vi "Lab 3 - Monty Hall - Copy (2).vi"() -> ()   [LabVIEW 2025]
panel:
  in  "Door 3":bool
  in  "Door 2":bool
  in  "Door 1":bool
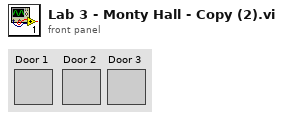
[diagram p1: front panel]
types:
  T1 = enum16{"Left Button", "Center Button", "Right Button", "Window Close"}
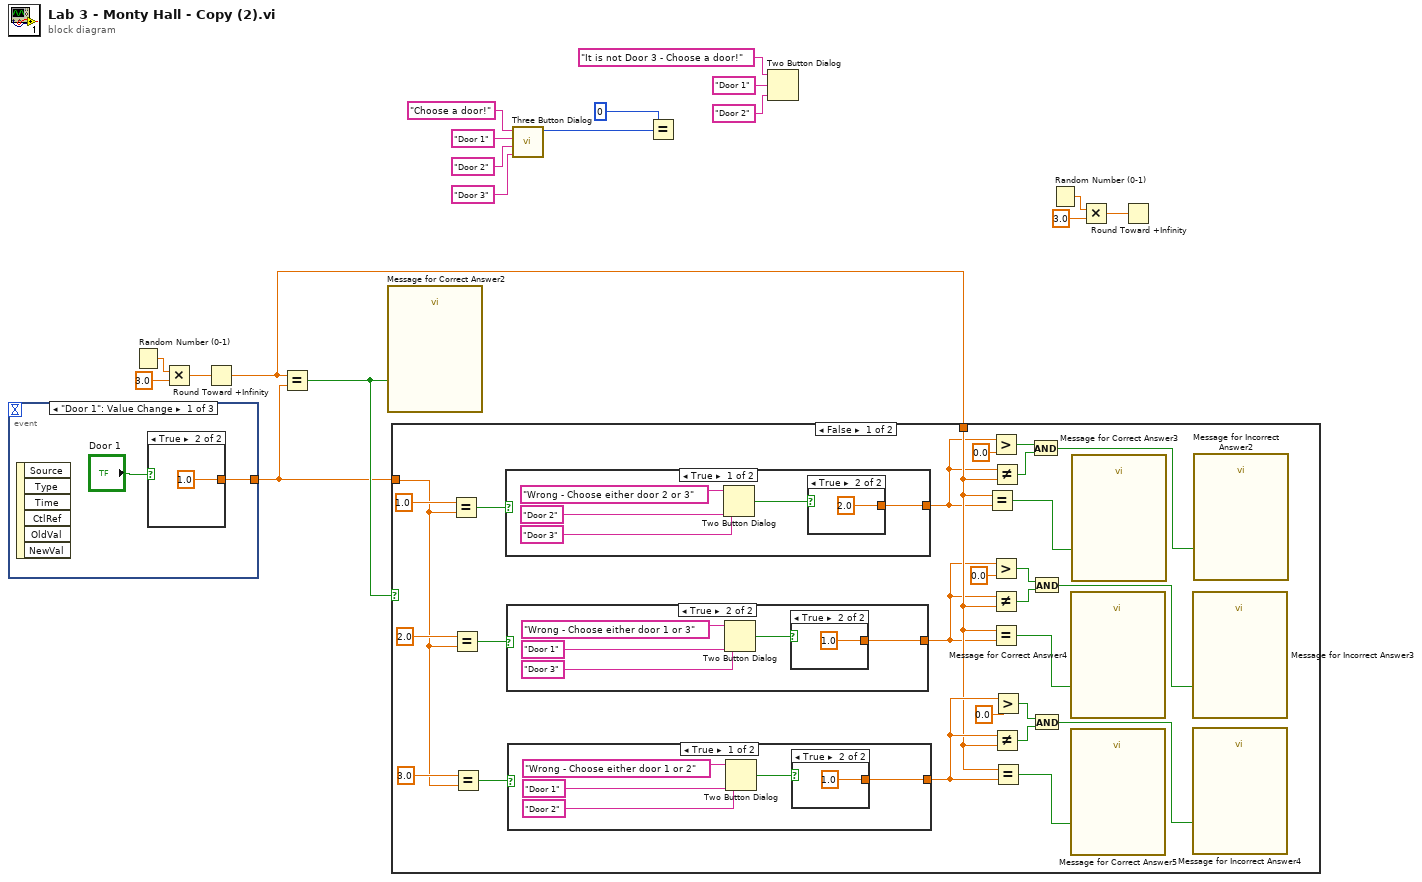
[diagram p0: block diagram]
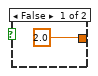
[diagram p2: hidden frame]
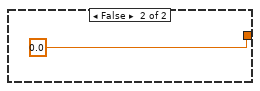
[diagram p3: hidden frame]
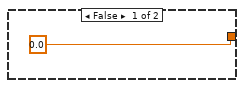
[diagram p4: hidden frame]
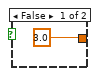
[diagram p5: hidden frame]
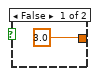
[diagram p6: hidden frame]
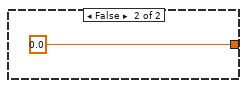
[diagram p7: hidden frame]
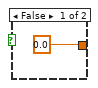
[diagram p9: hidden frame]
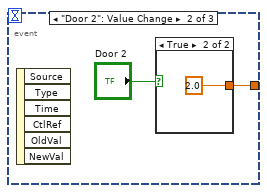
[diagram p10: hidden frame]
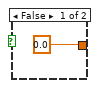
[diagram p11: hidden frame]
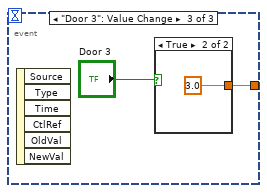
[diagram p12: hidden frame]
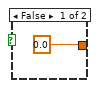
[diagram p13: hidden frame]
diagram:
  n1 = event shown="[0] \"Door 1\": Value Change" {
    selector: _ -> [_ _ _]
    dyn-events: _ -> [_ _ _]
    timeout: _ -> [_ _ _]
    tunnel: [w19 w23 w27] -> w15
    event "Door 1": Value Change {
      n2 = event-data() -> ()  [unwired: 1 in, 6 out]
      n3 = case shown="True" "Door 1" {
        tunnel: [0.0 1.0] -> w19
        frame False {
        }
        frame True {
        }
      }
    }
    event "Door 2": Value Change {
      n4 = event-data() -> ()  [unwired: 1 in, 6 out]
      n5 = case shown="True" "Door 2" {
        tunnel: [0.0 2.0] -> w23
        frame False {
        }
        frame True {
        }
      }
    }
    event "Door 3": Value Change {
      n6 = event-data() -> ()  [unwired: 1 in, 6 out]
      n7 = case shown="True" "Door 3" {
        tunnel: [0.0 3.0] -> w27
        frame False {
        }
        frame True {
        }
      }
    }
  }
  n8 = Random Number (0-1)() -> (number: 0 to 1=w17:dbl)
  n9 = Multiply(x=w17, y=3.0) -> (x*y=w14:dbl)
  n10 = Round Toward +Infinity(x=w14) -> (ceil(x): smallest int >= x=w13:dbl)
  n11 = Equal?(x=w13, y=w15) -> (x = y?=w16:bool)
  n12 = call "Message for Correct Answer2"("Enable"=w16) -> ()  [unwired: 9 in, 2 out]
  n13 = case shown="False" w16 {
    tunnel: w15 -> [w50 _]
    tunnel: w13 -> [w37 _]
    frame False {
      n14 = Equal?(x=1.0, y=w50) -> (x = y?=w53:bool)
      n15 = Equal?(x=2.0, y=w50) -> (x = y?=w51:bool)
      n16 = Equal?(x=3.0, y=w50) -> (x = y?=w52:bool)
      n17 = case shown="True" w53 {
        tunnel: [w73 0.0] -> w36
        frame True {
          n18 = Two Button Dialog(message="Wrong - Choose either door 2 or 3", 1:"Door 3", 2:"Door 2") -> (T button?=w74:bool)
          n19 = case shown="True" w74 {
            tunnel: [3.0 2.0] -> w73
            frame False {
            }
            frame True {
            }
          }
        }
        frame False {
        }
      }
      n20 = case shown="True" w51 {
        tunnel: [0.0 w66] -> w35
        frame False {
        }
        frame True {
          n21 = Two Button Dialog(message="Wrong - Choose either door 1 or 3", 1:"Door 3", 2:"Door 1") -> (T button?=w67:bool)
          n22 = case shown="True" w67 {
            tunnel: [3.0 1.0] -> w66
            frame False {
            }
            frame True {
            }
          }
        }
      }
      n23 = case shown="True" w52 {
        tunnel: [w57 0.0] -> w40
        frame True {
          n24 = Two Button Dialog(message="Wrong - Choose either door 1 or 2", 1:"Door 2", 2:"Door 1") -> (T button?=w58:bool)
          n25 = case shown="True" w58 {
            tunnel: [2.0 1.0] -> w57
            frame False {
            }
            frame True {
            }
          }
        }
        frame False {
        }
      }
      n26 = Equal?(x=w37, y=w36) -> (x = y?=w49:bool)
      n27 = Greater?(x=w36, y=0.0) -> (0:w33:bool)
      n28 = Greater?(x=w35, y=0.0) -> (0:w38:bool)
      n29 = Not Equal?(x=w35, y=w37) -> (x != y?=w39:bool)
      n30 = Equal?(x=w37, y=w35) -> (x = y?=w48:bool)
      n31 = Not Equal?(x=w36, y=w37) -> (x != y?=w34:bool)
      n32 = Not Equal?(x=w40, y=w37) -> (x != y?=w41:bool)
      n33 = Greater?(x=w40, y=0.0) -> (0:w43:bool)
      n34 = Equal?(x=w37, y=w40) -> (x = y?=w47:bool)
      n35 = And(x=w33, y=w34) -> (x .and. y?=w32:bool)
      n36 = And(x=w38, y=w39) -> (x .and. y?=w31:bool)
      n37 = And(x=w43, y=w41) -> (x .and. y?=w42:bool)
      n38 = call "Message for Correct Answer4"("Enable"=w48) -> ()  [unwired: 9 in, 2 out]
      n39 = call "Message for Correct Answer5"("Enable"=w47) -> ()  [unwired: 9 in, 2 out]
      n40 = call "Message for Correct Answer3"("Enable"=w49) -> ()  [unwired: 9 in, 2 out]
      n41 = call "Message for Incorrect Answer3"("Enable"=w31) -> ()  [unwired: 9 in, 2 out]
      n42 = call "Message for Incorrect Answer4"("Enable"=w42) -> ()  [unwired: 9 in, 2 out]
      n43 = call "Message for Incorrect Answer2"("Enable"=w32) -> ()  [unwired: 9 in, 2 out]
    }
    frame True {
    }
  }
  n44 = call <vilib>:"Three Button Dialog.vi"("Right Button Text (\"Cancel\")"="Door 3", "Center Button Text (\"No\")"="Door 2", "Left Button Text (\"Yes\")"="Door 1", "message"="Choose a door!") -> ("Which Button?"=w2:T1)  [unwired: 7 in]
  n45 = Equal?(x=0, y=w2) -> ()  [unwired: 1 out]
  n46 = Two Button Dialog(message="It is not Door 3 - Choose a door!", 1:"Door 2", 2:"Door 1") -> ()  [unwired: 1 out]
  n47 = Random Number (0-1)() -> (number: 0 to 1=w4:dbl)
  n48 = Multiply(x=w4, y=3.0) -> (x*y=w3:dbl)
  n49 = Round Toward +Infinity(x=w3) -> ()  [unwired: 1 out]
